vi "RFmx_Cntr_Fetch_Result.vi"(6 "RFmx_Data_In":refnum<queue>, 7 "Meas_Type":string[](array[string])=["ACP"], 8 "error in (no error)":errorcluster, 11 "Instrument Handle in":refnum<k21>="VST") -> (0 "error out":errorcluster, 3 "Instrument Handle out":refnum<k21>="VST")   [LabVIEW 2014]
uses:
  02_Controls/Message_Data_Ctl.ctl
  <vilib>/RFmx/RFInstr/mx/RFmxInstr.llb/RFmxInstr Build Signal String.vi
  <vilib>/RFmx/SpecAn/mx/RFmxSpecAn.llb/RFmxSpecAn ACP Fetch Total Carrier Power.vi
  <vilib>/RFmx/SpecAn/mx/RFmxSpecAn.llb/RFmxSpecAn ACP Fetch Offset Measurement (Array).vi
  <vilib>/RFmx/SpecAn/mx/RFmxSpecAn.llb/RFmxSpecAn CHP Fetch Total Carrier Power.vi
  <vilib>/RFmx/SpecAn/mx/RFmxSpecAn.llb/RFmxSpecAn FCnt Fetch Measurement.vi
  <vilib>/RFmx/SpecAn/mx/RFmxSpecAn.llb/RFmxSpecAn OBW Fetch Measurement.vi
  <vilib>/RFmx/SpecAn/mx/RFmxSpecAn.llb/RFmxSpecAn TXP Fetch Measurement.vi
  <vilib>/RFmx/SpecAn/mx/RFmxSpecAn.llb/RFmxSpecAn TXP Fetch Power Trace.vi
  <vilib>/RFmx/SpecAn/mx/RFmxSpecAn.llb/RFmxSpecAn CCDF Fetch Power.vi
  <vilib>/RFmx/SpecAn/mx/RFmxSpecAn.llb/RFmxSpecAn CCDF Fetch Probabilities Trace.vi
  <vilib>/RFmx/SpecAn/mx/RFmxSpecAn.llb/RFmxSpecAn CCDF Fetch Gaussian Probabilities Trace.vi
  <vilib>/RFmx/SpecAn/mx/RFmxSpecAn.llb/RFmxSpecAn Spectrum Fetch Spectrum.vi
  <vilib>/RFmx/SpecAn/mx/RFmxSpecAn.llb/RFmxSpecAn Spectrum Fetch Measurement.vi
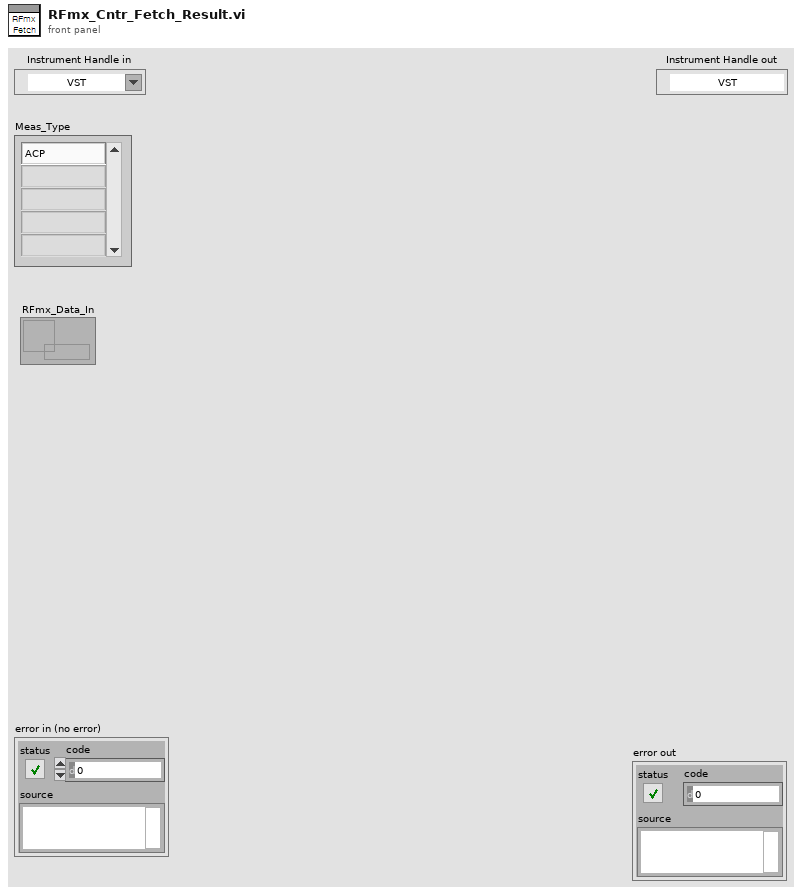
[diagram p1: front panel]
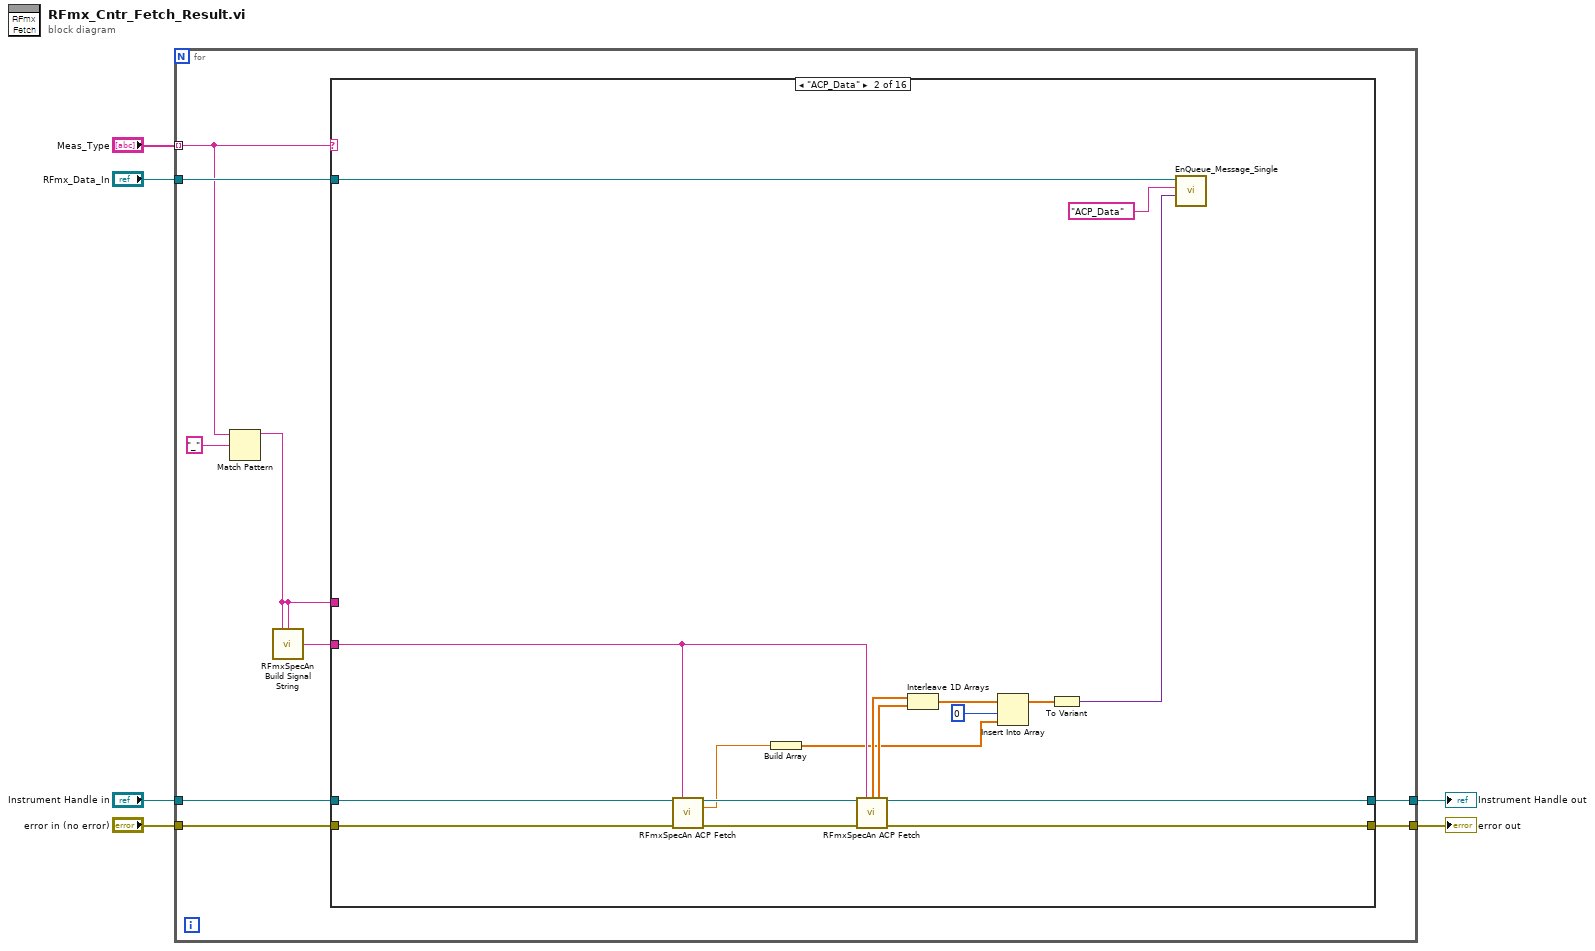
[diagram p0: block diagram]
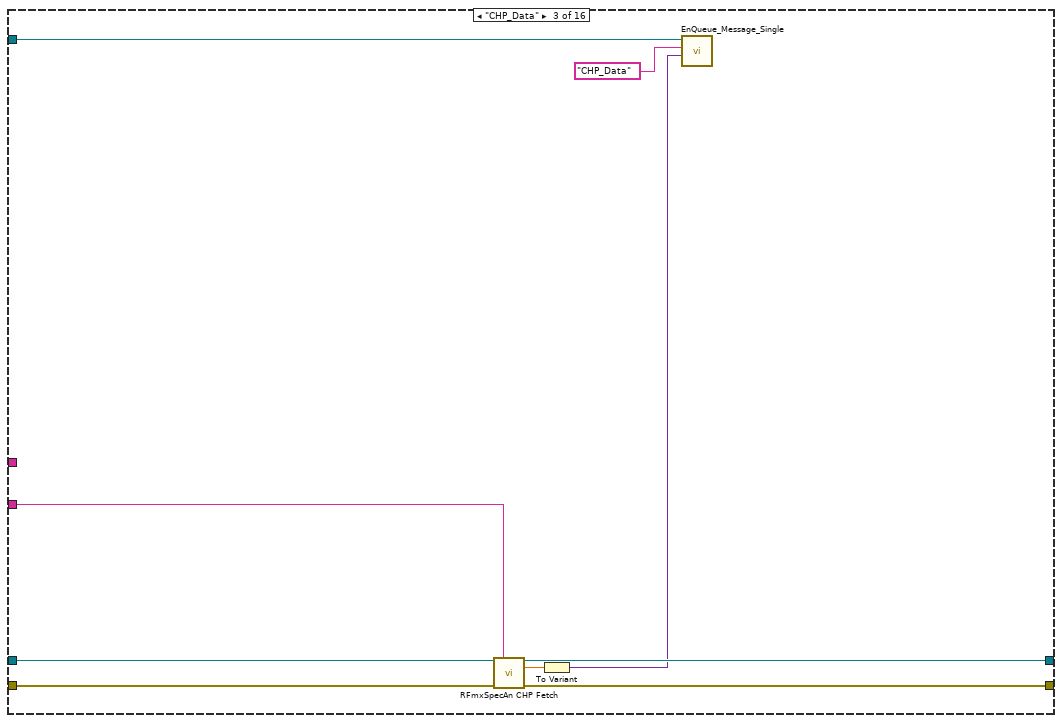
[diagram p3: hidden frame]
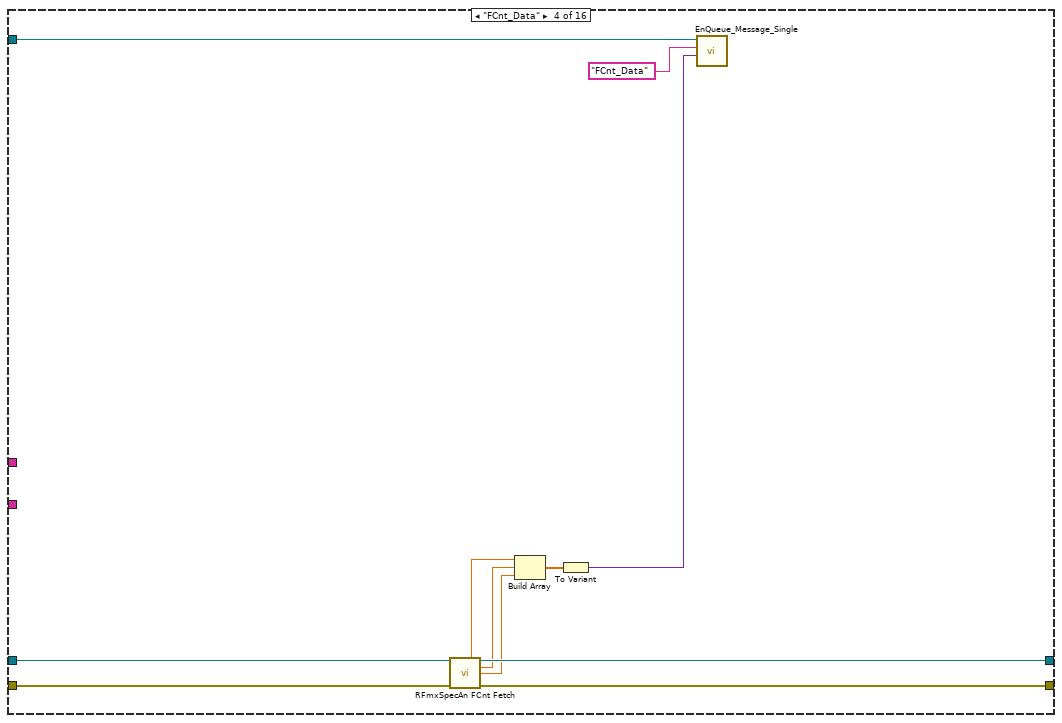
[diagram p4: hidden frame]
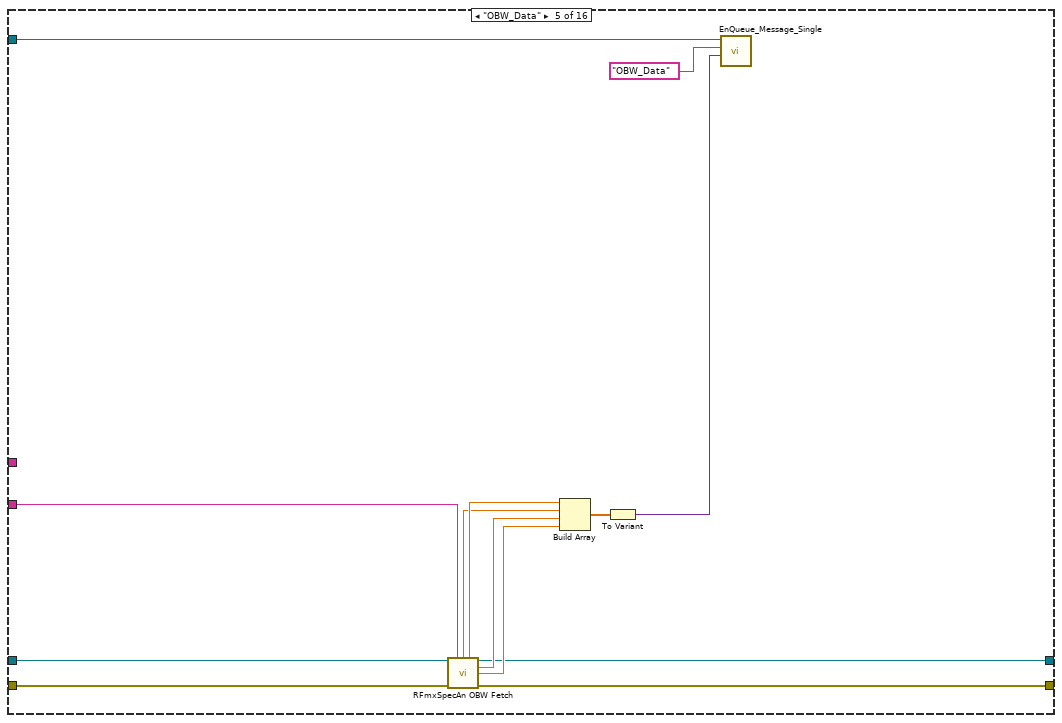
[diagram p5: hidden frame]
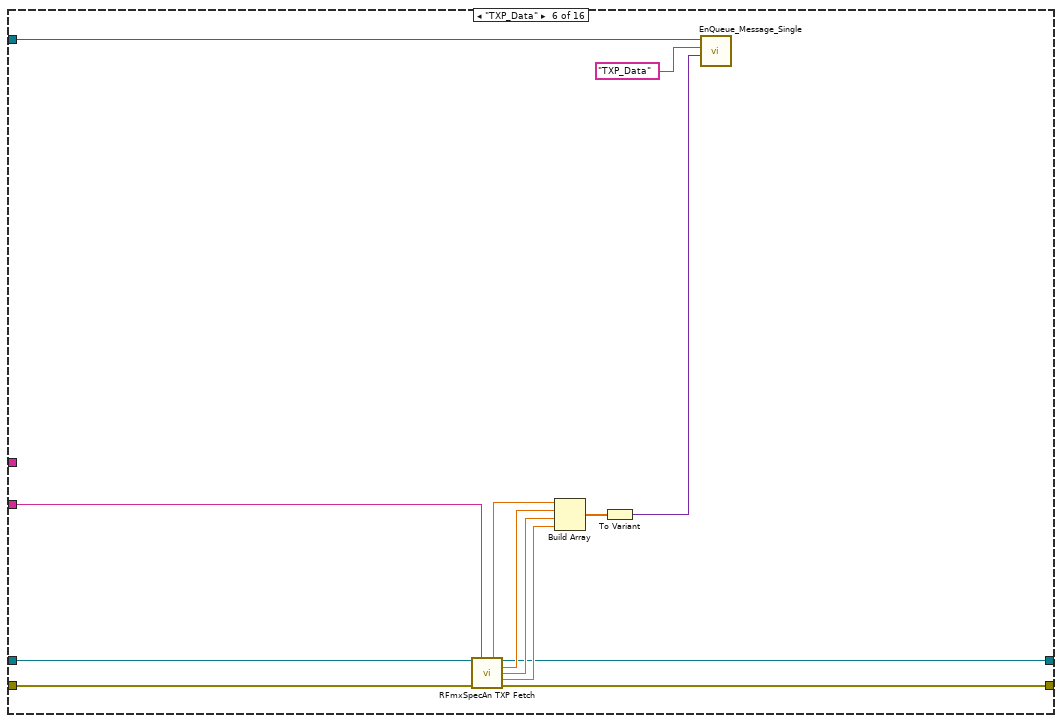
[diagram p6: hidden frame]
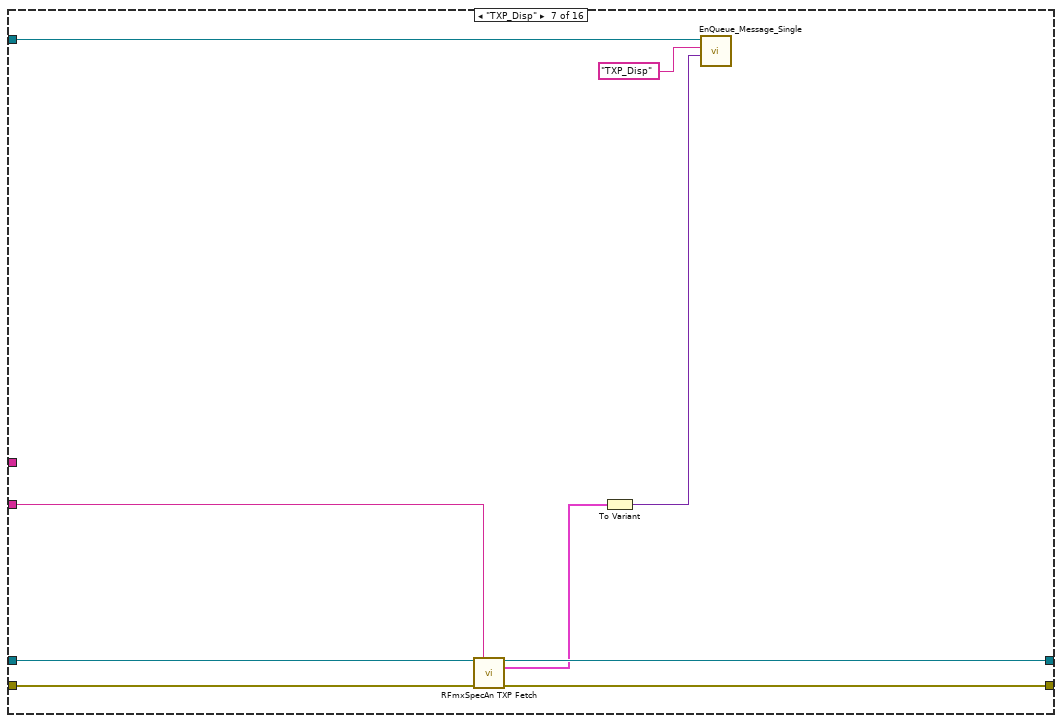
[diagram p7: hidden frame]
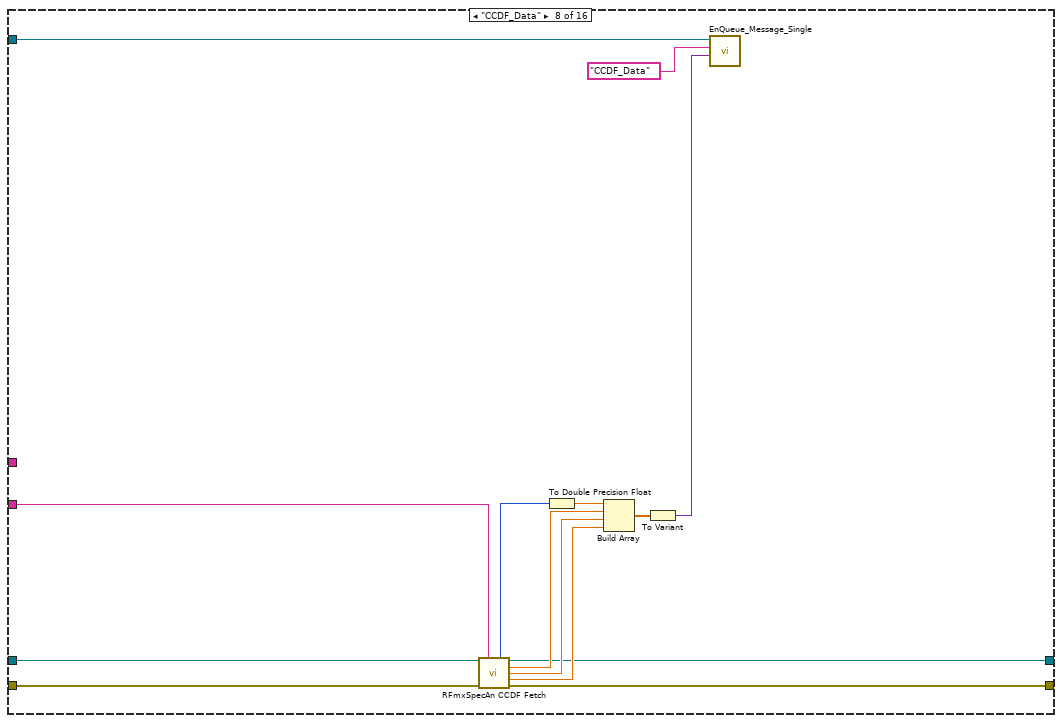
[diagram p8: hidden frame]
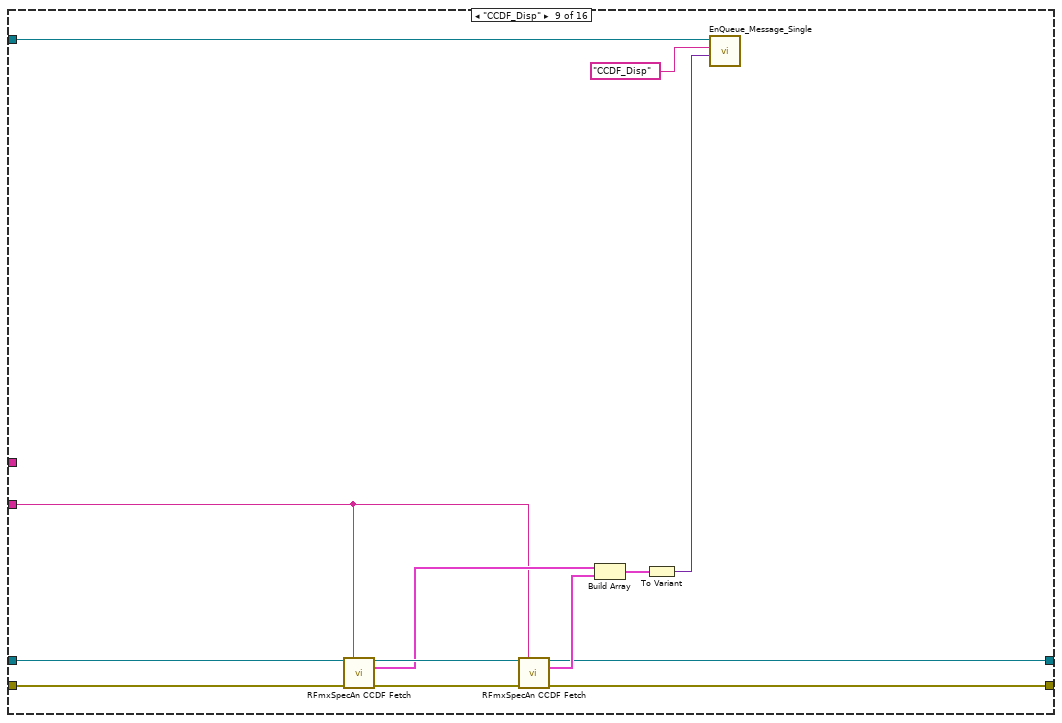
[diagram p9: hidden frame]
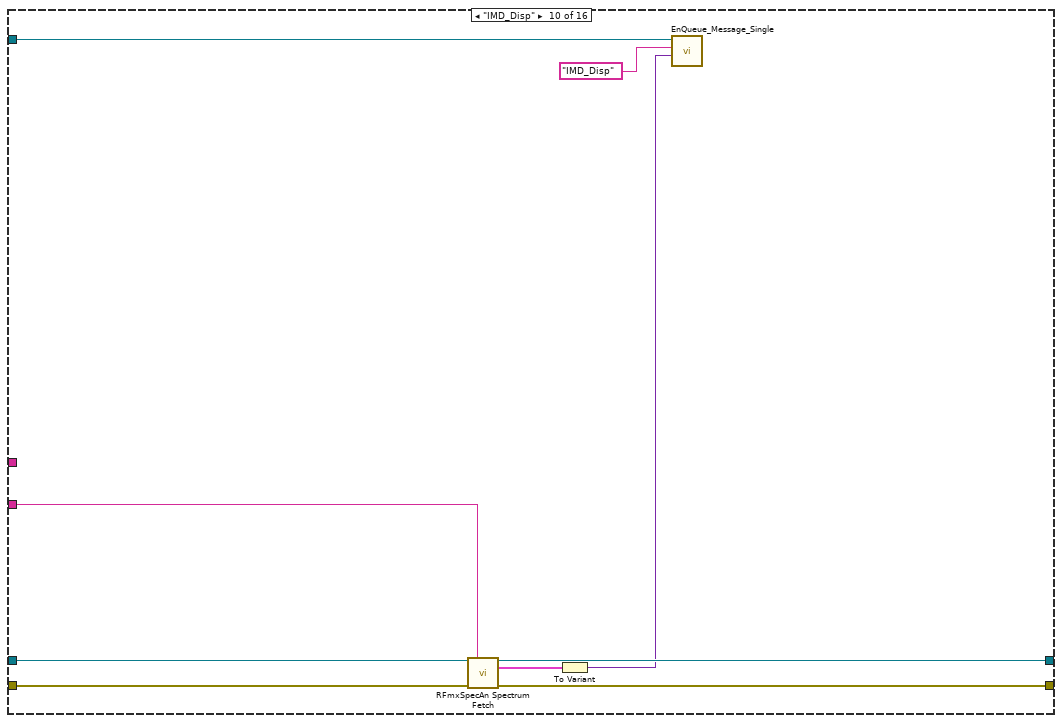
[diagram p10: hidden frame]
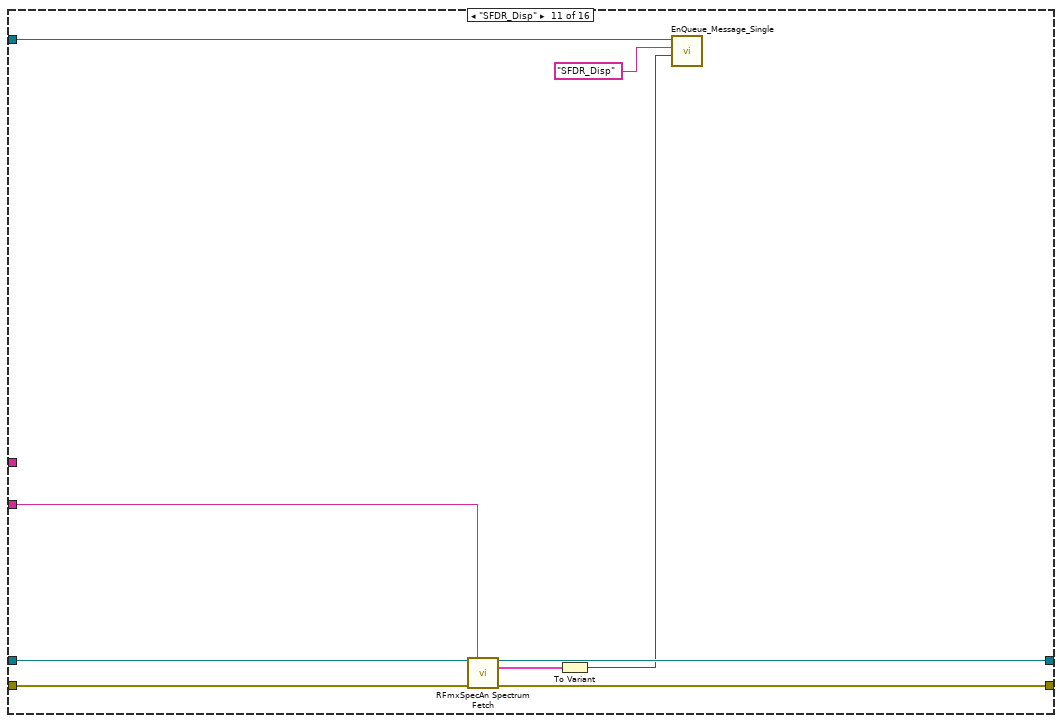
[diagram p11: hidden frame]
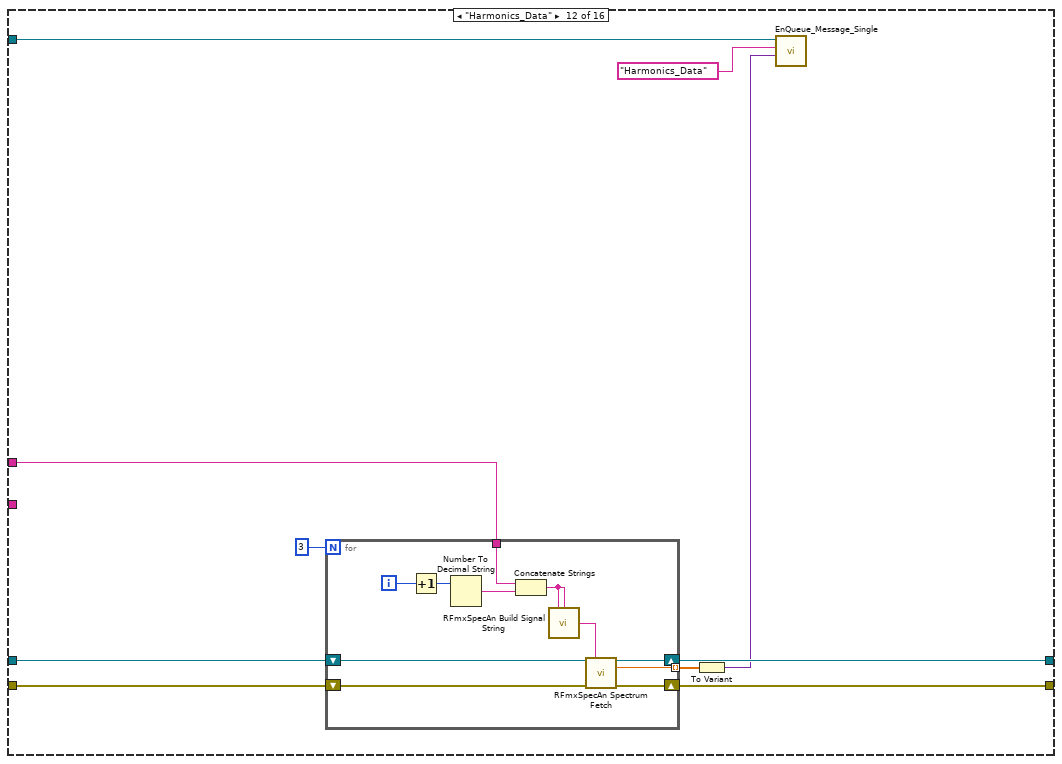
[diagram p12: hidden frame]
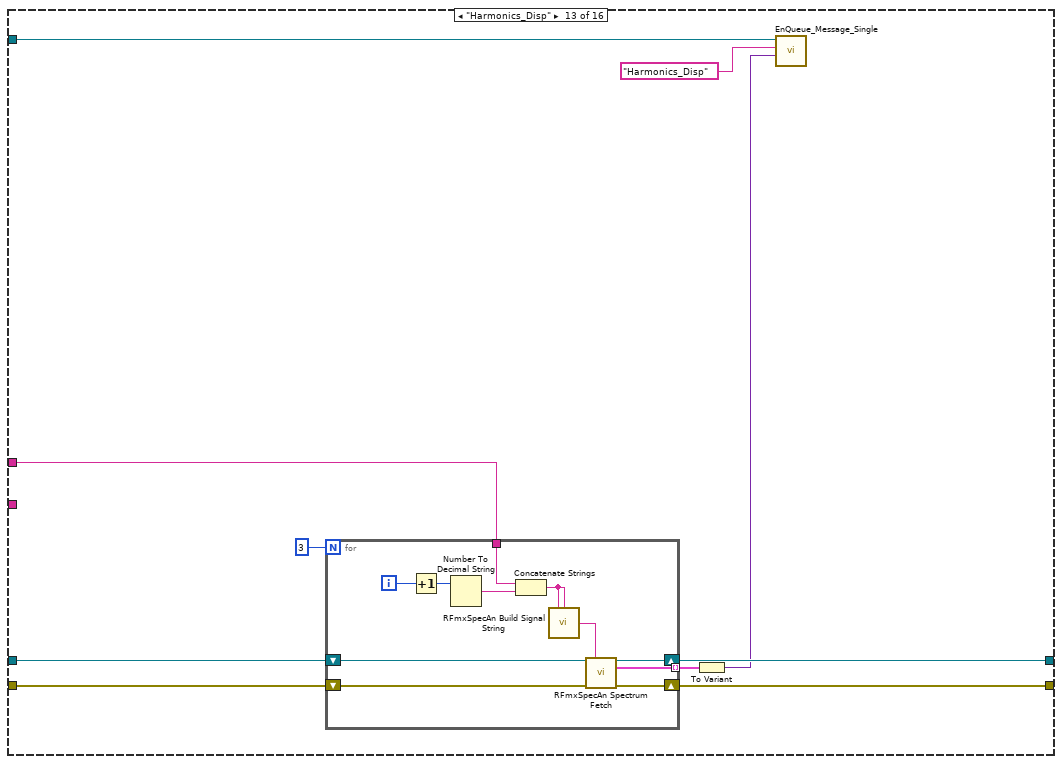
[diagram p13: hidden frame]
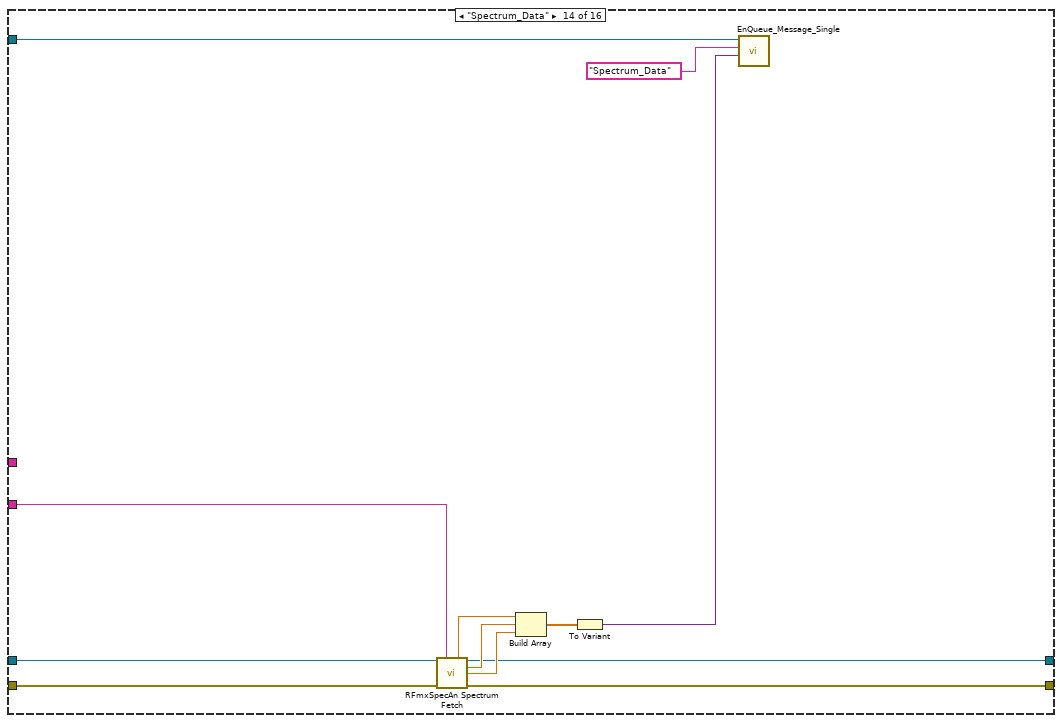
[diagram p14: hidden frame]
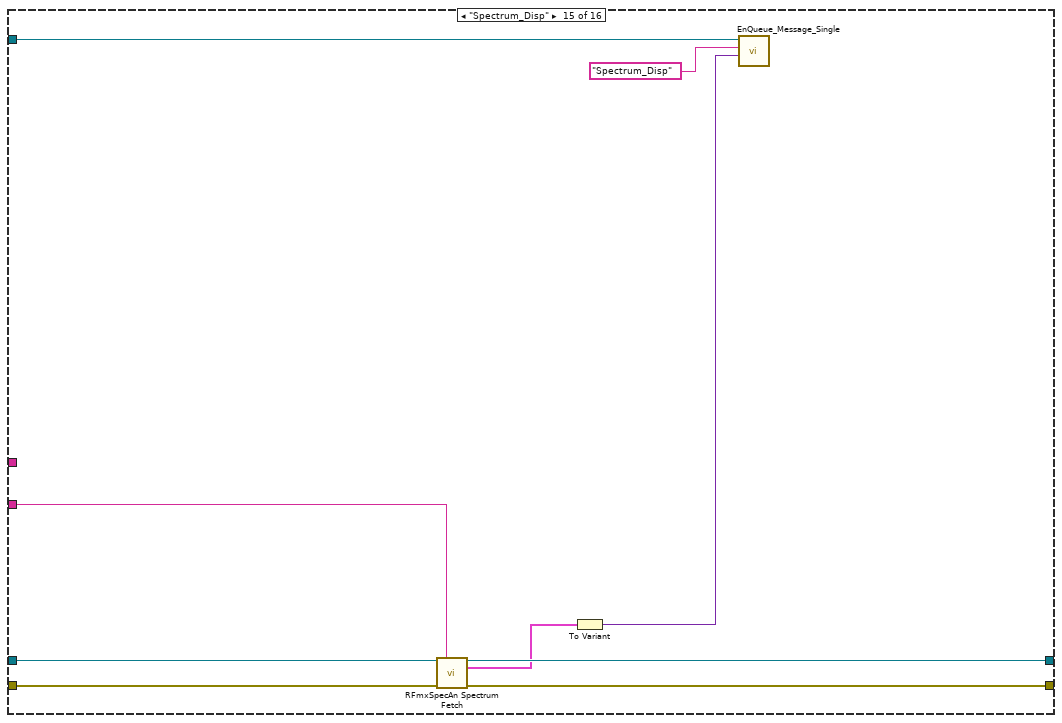
[diagram p15: hidden frame]
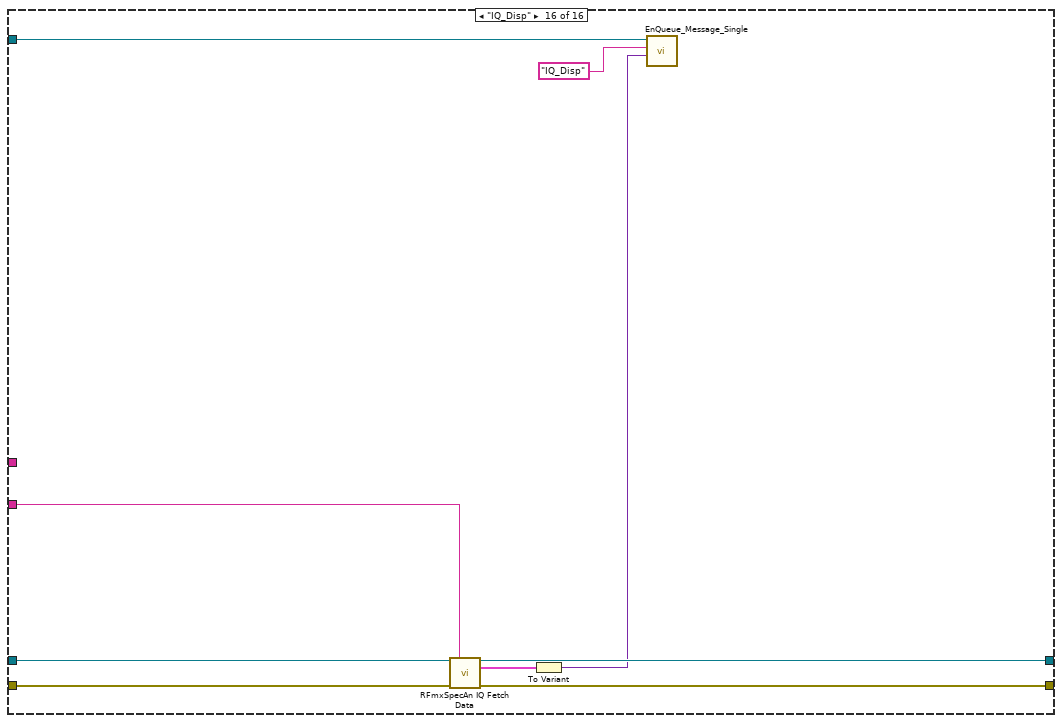
[diagram p16: hidden frame]
diagram:
  n1 = for {
    tunnel: [w15] -> w6
    tunnel: [w14] -> w5
    tunnel: "Meas_Type" -> [w8] mode=indexing
    tunnel: "Instrument Handle in" -> [w12]
    tunnel: "error in (no error)" -> [w11]
    tunnel: "RFmx_Data_In" -> [w10]
    n2 = Match Pattern(string=w8, regular expression="_") -> (before substring=w7:string)  [unwired: 1 in, 3 out]
    n3 = call <vilib>:"RFmxSpecAn Build Signal String.vi"("Signal Name"=w7, "Result Name"=w7) -> ("Selector String"=w13:string)  [unwired: 13 in]
    n4 = case shown="\"ACP_Data\"" w8 {
      tunnel: [w17 w22 w41 w52 w61 w69 w83 w95 w108 w123 w132 w140 w161 w183 w195 w200] -> w14
      tunnel: [w16 w21 w40 w51 w60 w68 w84 w94 w107 w122 w131 w139 w160 w182 w194 w199] -> w15
      tunnel: w13 -> [_ w23 w35 _ w59 w74 w81 w96 w104 w121 w130 _ _ w177 w189 w204]
      tunnel: w7 -> [_ _ _ _ _ _ _ _ _ _ _ w141 w162 _ _ _]
      tunnel: w12 -> [w17 w28 w43 w54 w63 w76 w86 w98 w110 w125 w134 w143 w164 w185 w197 w206]
      tunnel: w11 -> [w16 w27 w42 w53 w62 w75 w85 w97 w109 w124 w133 w142 w163 w184 w196 w205]
      tunnel: w10 -> [_ w20 w38 w45 w57 w71 w88 w92 w115 w119 w128 w137 w158 w180 w192 w202]
      frame "Nothing", Default {
      }
      frame "ACP_Data" {
        n5 = call-poly <vilib>:"RFmxSpecAn ACP Fetch.vi"("Instrument Handle In"=w28, "Selector String"=w23, "error in (no error)"=w27) -> ("Instrument Handle Out"=w34:refnum<k21>, "Total Carrier Power (dBm or dBm/Hz)"=w30:dbl, "error out"=w33:errorcluster)  [unwired: 10 in]
        n6 = Build Array(w30) -> (w18:dbl[])
        n7 = call-poly <vilib>:"RFmxSpecAn ACP Fetch.vi"("Instrument Handle In"=w34, "Selector String"=w23, "error in (no error)"=w33) -> ("Lower Absolute Power (dBm or dBm/Hz)"=w32:dbl[], "Upper Absolute Power (dBm or dBm/Hz)"=w31:dbl[], "Instrument Handle Out"=w22:refnum<k21>, "error out"=w21:errorcluster)  [unwired: 7 in, 2 out]
        n8 = Interleave 1D Arrays(w32, w31) -> (w19:dbl[])
        n9 = Insert Into Array(array=w19, index=0, new element=w18) -> (w24:dbl[])
        n10 = To Variant(anything=w24) -> (Variant=w26:variant)
        n11 = call "EnQueue_Message_Single.vi"("Message Data"=w26, "Message"="ACP_Data", "Message_Queue"=w20) -> ()  [unwired: 7 in, 2 out]
      }
      frame "CHP_Data" {
        n12 = call-poly <vilib>:"RFmxSpecAn CHP Fetch.vi"("Instrument Handle In"=w43, "Selector String"=w35, "error in (no error)"=w42) -> ("Instrument Handle Out"=w41:refnum<k21>, "Total Carrier Power (dBm)"=w37:dbl, "error out"=w40:errorcluster)  [unwired: 10 in]
        n13 = To Variant(anything=w37) -> (Variant=w36:variant)
        n14 = call "EnQueue_Message_Single.vi"("Message Data"=w36, "Message"="CHP_Data", "Message_Queue"=w38) -> ()  [unwired: 7 in, 2 out]
      }
      frame "FCnt_Data" {
        n15 = call-poly <vilib>:"RFmxSpecAn FCnt Fetch.vi"("Instrument Handle In"=w54, "error in (no error)"=w53) -> ("Average Absolute Frequency (Hz)"=w50:dbl, "Instrument Handle Out"=w52:refnum<k21>, "Average Relative Frequency (Hz)"=w49:dbl, "Mean Phase (deg)"=w48:dbl, "error out"=w51:errorcluster)  [unwired: 9 in]
        n16 = Build Array(w50, w49, w48) -> (w47:dbl[])
        n17 = To Variant(anything=w47) -> (Variant=w44:variant)
        n18 = call "EnQueue_Message_Single.vi"("Message Data"=w44, "Message"="FCnt_Data", "Message_Queue"=w45) -> ()  [unwired: 7 in, 2 out]
      }
      frame "OBW_Data" {
        n19 = call-poly <vilib>:"RFmxSpecAn OBW Fetch.vi"("Instrument Handle In"=w63, "Selector String"=w59, "error in (no error)"=w62) -> ("Stop Frequency (Hz)"=w66:dbl, "Start Frequency (Hz)"=w67:dbl, "Instrument Handle Out"=w61:refnum<k21>, "Occupied Bandwidth (Hz)"=w65:dbl, "Average Power (dBm or dBm/Hz)"=w64:dbl, "error out"=w60:errorcluster)  [unwired: 6 in, 1 out]
        n20 = Build Array(w67, w66, w65, w64) -> (w58:dbl[])
        n21 = To Variant(anything=w58) -> (Variant=w56:variant)
        n22 = call "EnQueue_Message_Single.vi"("Message Data"=w56, "Message"="OBW_Data", "Message_Queue"=w57) -> ()  [unwired: 7 in, 2 out]
      }
      frame "TXP_Data" {
        n23 = call-poly <vilib>:"RFmxSpecAn TXP Fetch.vi"("Instrument Handle In"=w76, "Selector String"=w74, "error in (no error)"=w75) -> ("Minimum Power (dBm)"=w80:dbl, "Instrument Handle Out"=w69:refnum<k21>, "Average Mean Power (dBm)"=w79:dbl, "Peak to Average Ratio (dB)"=w78:dbl, "Maximum Power (dBm)"=w77:dbl, "error out"=w68:errorcluster)  [unwired: 7 in]
        n24 = Build Array(w80, w79, w78, w77) -> (w73:dbl[])
        n25 = To Variant(anything=w73) -> (Variant=w70:variant)
        n26 = call "EnQueue_Message_Single.vi"("Message Data"=w70, "Message"="TXP_Data", "Message_Queue"=w71) -> ()  [unwired: 7 in, 2 out]
      }
      frame "TXP_Disp" {
        n27 = call-poly <vilib>:"RFmxSpecAn TXP Fetch.vi"("Instrument Handle In"=w86, "Selector String"=w81, "error in (no error)"=w85) -> ("Instrument Handle Out"=w83:refnum<k21>, "Power (dBm)"=w82:cluster{"x0":dbl, "dx":dbl, "y":sgl[]}, "error out"=w84:errorcluster)  [unwired: 10 in]
        n28 = To Variant(anything=w82) -> (Variant=w87:variant)
        n29 = call "EnQueue_Message_Single.vi"("Message Data"=w87, "Message"="TXP_Disp", "Message_Queue"=w88) -> ()  [unwired: 7 in, 2 out]
      }
      frame "CCDF_Data" {
        n30 = call-poly <vilib>:"RFmxSpecAn CCDF Fetch.vi"("Instrument Handle In"=w98, "Selector String"=w96, "error in (no error)"=w97) -> ("Measured Samples Count"=w100:i32, "Instrument Handle Out"=w95:refnum<k21>, "Mean Power (dBm)"=w103:dbl, "Mean Power Percentile (%)"=w102:dbl, "Peak Power (dB)"=w101:dbl, "error out"=w94:errorcluster)  [unwired: 7 in]
        n31 = To Double Precision Float(number=w100) -> (double precision float=w99:dbl)
        n32 = Build Array(w99, w103, w102, w101) -> (w91:dbl[])
        n33 = To Variant(anything=w91) -> (Variant=w90:variant)
        n34 = call "EnQueue_Message_Single.vi"("Message Data"=w90, "Message"="CCDF_Data", "Message_Queue"=w92) -> ()  [unwired: 7 in, 2 out]
      }
      frame "CCDF_Disp" {
        n35 = call-poly <vilib>:"RFmxSpecAn CCDF Fetch.vi"("Instrument Handle In"=w110, "Selector String"=w104, "error in (no error)"=w109) -> ("Instrument Handle Out"=w113:refnum<k21>, "Probabilities (%)"=w112:cluster{"x0":dbl, "dx":dbl, "y":sgl[]}, "error out"=w114:errorcluster)  [unwired: 10 in]
        n36 = call-poly <vilib>:"RFmxSpecAn CCDF Fetch.vi"("Instrument Handle In"=w113, "Selector String"=w104, "error in (no error)"=w114) -> ("Instrument Handle Out"=w108:refnum<k21>, "Gaussian Probabilities (%)"=w111:cluster{"x0":dbl, "dx":dbl, "y":sgl[]}, "error out"=w107:errorcluster)  [unwired: 10 in]
        n37 = Build Array(w112, w111) -> (w106:cluster{"x0":dbl, "dx":dbl, "y":sgl[]}[])
        n38 = To Variant(anything=w106) -> (Variant=w105:variant)
        n39 = call "EnQueue_Message_Single.vi"("Message Data"=w105, "Message"="CCDF_Disp", "Message_Queue"=w115) -> ()  [unwired: 7 in, 2 out]
      }
      frame "IMD_Disp" {
        n40 = call-poly <vilib>:"RFmxSpecAn Spectrum Fetch.vi"("Instrument Handle In"=w125, "Selector String"=w121, "error in (no error)"=w124) -> ("Instrument Handle Out"=w123:refnum<k21>, "Spectrum"=w118:cluster{"x0":dbl, "dx":dbl, "y":sgl[]}, "error out"=w122:errorcluster)  [unwired: 10 in]
        n41 = To Variant(anything=w118) -> (Variant=w117:variant)
        n42 = call "EnQueue_Message_Single.vi"("Message Data"=w117, "Message"="IMD_Disp", "Message_Queue"=w119) -> ()  [unwired: 7 in, 2 out]
      }
      frame "SFDR_Disp" {
        n43 = call-poly <vilib>:"RFmxSpecAn Spectrum Fetch.vi"("Instrument Handle In"=w134, "Selector String"=w130, "error in (no error)"=w133) -> ("Instrument Handle Out"=w132:refnum<k21>, "Spectrum"=w127:cluster{"x0":dbl, "dx":dbl, "y":sgl[]}, "error out"=w131:errorcluster)  [unwired: 10 in]
        n44 = To Variant(anything=w127) -> (Variant=w126:variant)
        n45 = call "EnQueue_Message_Single.vi"("Message Data"=w126, "Message"="SFDR_Disp", "Message_Queue"=w128) -> ()  [unwired: 7 in, 2 out]
      }
      frame "Harmonics_Data" {
        n46 = for {
          N: 3 -> [_]
          shift-right: [w150] -> w140
          shift-left: w143 -> [w155]
          shift-right: [w149] -> w139
          shift-left: w142 -> [w154]
          tunnel: [w148] -> w136 mode=indexing
          tunnel: w141 -> [w145]
          i -> [w147]
          n47 = Increment(x=w147) -> (x+1=w146:i32)
          n48 = Number To Decimal String(number=w146) -> (decimal integer string=w152:string)  [unwired: 1 in]
          n49 = Concatenate Strings(w145, w152) -> (w153:string)
          n50 = call <vilib>:"RFmxSpecAn Build Signal String.vi"("Signal Name"=w153, "Result Name"=w153) -> ("Selector String"=w151:string)  [unwired: 13 in]
          n51 = call-poly <vilib>:"RFmxSpecAn Spectrum Fetch.vi"("Instrument Handle In"=w155, "Selector String"=w151, "error in (no error)"=w154) -> ("Instrument Handle Out"=w150:refnum<k21>, "Peak Amplitude"=w148:dbl, "error out"=w149:errorcluster)  [unwired: 8 in, 2 out]
        }
        n52 = To Variant(anything=w136) -> (Variant=w135:variant)
        n53 = call "EnQueue_Message_Single.vi"("Message Data"=w135, "Message"="Harmonics_Data", "Message_Queue"=w137) -> ()  [unwired: 7 in, 2 out]
      }
      frame "Harmonics_Disp" {
        n54 = for {
          N: 3 -> [_]
          shift-right: [w171] -> w161
          shift-left: w164 -> [w176]
          shift-right: [w170] -> w160
          shift-left: w163 -> [w175]
          tunnel: [w169] -> w157 mode=indexing
          tunnel: w162 -> [w166]
          i -> [w168]
          n55 = Increment(x=w168) -> (x+1=w167:i32)
          n56 = Number To Decimal String(number=w167) -> (decimal integer string=w173:string)  [unwired: 1 in]
          n57 = Concatenate Strings(w166, w173) -> (w174:string)
          n58 = call <vilib>:"RFmxSpecAn Build Signal String.vi"("Signal Name"=w174, "Result Name"=w174) -> ("Selector String"=w172:string)  [unwired: 13 in]
          n59 = call-poly <vilib>:"RFmxSpecAn Spectrum Fetch.vi"("Instrument Handle In"=w176, "Selector String"=w172, "error in (no error)"=w175) -> ("Instrument Handle Out"=w171:refnum<k21>, "Spectrum"=w169:cluster{"x0":dbl, "dx":dbl, "y":sgl[]}, "error out"=w170:errorcluster)  [unwired: 10 in]
        }
        n60 = To Variant(anything=w157) -> (Variant=w156:variant)
        n61 = call "EnQueue_Message_Single.vi"("Message Data"=w156, "Message"="Harmonics_Disp", "Message_Queue"=w158) -> ()  [unwired: 7 in, 2 out]
      }
      frame "Spectrum_Data" {
        n62 = call-poly <vilib>:"RFmxSpecAn Spectrum Fetch.vi"("Instrument Handle In"=w185, "Selector String"=w177, "error in (no error)"=w184) -> ("Frequency Resolution (Hz)"=w188:dbl, "Instrument Handle Out"=w183:refnum<k21>, "Peak Amplitude"=w187:dbl, "Peak Frequency (Hz)"=w186:dbl, "error out"=w182:errorcluster)  [unwired: 8 in]
        n63 = Build Array(w188, w187, w186) -> (w179:dbl[])
        n64 = To Variant(anything=w179) -> (Variant=w178:variant)
        n65 = call "EnQueue_Message_Single.vi"("Message Data"=w178, "Message"="Spectrum_Data", "Message_Queue"=w180) -> ()  [unwired: 7 in, 2 out]
      }
      frame "Spectrum_Disp" {
        n66 = call-poly <vilib>:"RFmxSpecAn Spectrum Fetch.vi"("Instrument Handle In"=w197, "Selector String"=w189, "error in (no error)"=w196) -> ("Instrument Handle Out"=w195:refnum<k21>, "Spectrum"=w190:cluster{"x0":dbl, "dx":dbl, "y":sgl[]}, "error out"=w194:errorcluster)  [unwired: 10 in]
        n67 = To Variant(anything=w190) -> (Variant=w191:variant)
        n68 = call "EnQueue_Message_Single.vi"("Message Data"=w191, "Message"="Spectrum_Disp", "Message_Queue"=w192) -> ()  [unwired: 7 in, 2 out]
      }
      frame "IQ_Disp" {
        n69 = call <vilib>:"RFmxSpecAn IQ Fetch Data.vi"("Instrument Handle In"=w206, "Selector String"=w204, "error in (no error)"=w205) -> ("Instrument Handle Out"=w200:refnum<k21>, "Data"=w201:cluster{"t0":dbl, "dt":dbl, "Y":csg[]}, "error out"=w199:errorcluster)  [unwired: 10 in]
        n70 = To Variant(anything=w201) -> (Variant=w198:variant)
        n71 = call "EnQueue_Message_Single.vi"("Message Data"=w198, "Message"="IQ_Disp", "Message_Queue"=w202) -> ()  [unwired: 7 in, 2 out]
      }
    }
  }
  "Instrument Handle out" <- w5
  "error out" <- w6
